vi "DefBallPosSkillVSS.vi"(8 "error in (no error)":errorcluster, 11 "DefBallPosSkillVSS in":refnum<class "DefBallPosSkillVSS.lvclass">) -> (0 "error out":errorcluster, 3 "DefBallPosSkillVSS out":refnum<class "DefBallPosSkillVSS.lvclass">)   [LabVIEW 2018, in "DefBallPosSkillVSS.lvclass"]
uses:
  DefBallPosSkillVSS.lvclass
  Robot_class/Robot.lvclass
  Ball_class/Ball.lvclass
  C:/Users/duduw/Desktop/IME/roboime/teste simulador/SSL_AI/Object_class/Object.lvclass
  Object_class/Object.lvclass/Object.ctl
  Robot_class/Robot.lvclass/Robot.ctl
  Object_class/Read y.vi
  Robot_class/Write dest_y.vi
panel:
  out "Robot out":refnum<class "Robot.lvclass">
  in  "BallRef":refnum<class "Ball.lvclass">
  in  "Robot in":refnum<class "Robot.lvclass">
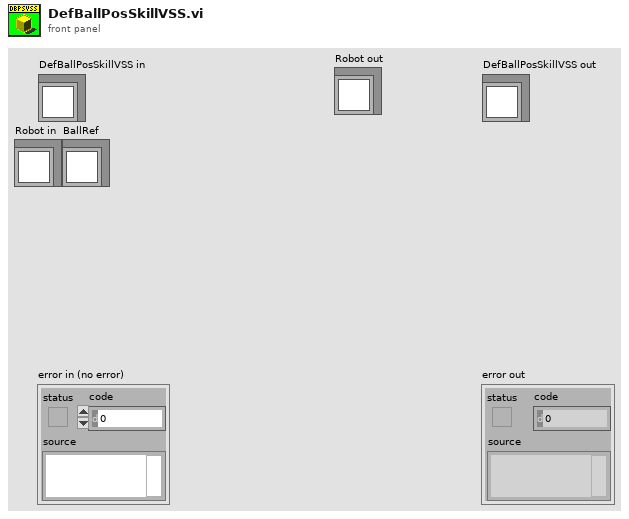
[diagram p1: front panel]
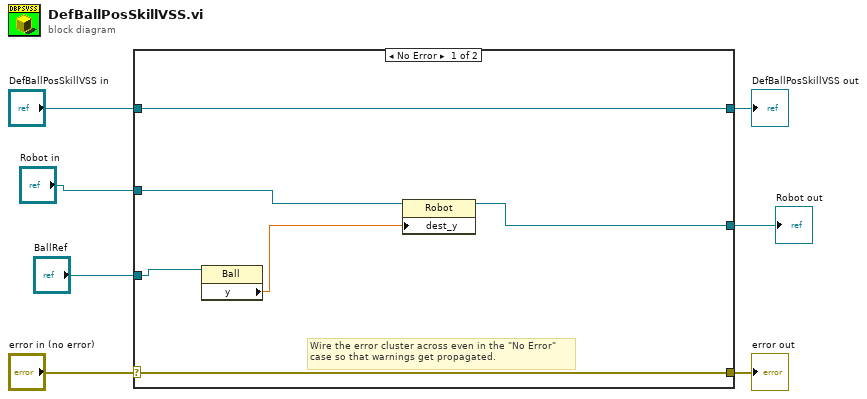
[diagram p0: block diagram]
diagram:
  n1 = case shown="No Error" "error in (no error)" {
    selector: "error in (no error)" -> [w12 w16]
    tunnel: [w12 w16] -> w6
    tunnel: [w13 w15] -> w4
    tunnel: "DefBallPosSkillVSS in" -> [w13 w15]
    tunnel: "Robot in" -> [w11 w14]
    tunnel: "BallRef" -> [w9 _]
    tunnel: [w10 w14] -> w1
    frame No Error {
      # "Wire the error cluster across even in the \"No Error\"\ncase so that warnings get propagated."
      n2 = property class="Ball"(reference=w9) -> ("y"=w8:dbl)  [unwired: 1 in, 2 out]
      n3 = property class="Robot"(reference=w11, "dest_y"=w8) -> (reference out=w10:refnum<class "Robot.lvclass">)  [unwired: 1 in, 1 out]
    }
    frame Error {
    }
  }
  "error out" <- w6
  "DefBallPosSkillVSS out" <- w4
  "Robot out" <- w1
